vi "Sample--SaveandReadData.vi"() -> ()   [LabVIEW 2013]
doc: "This samples demonstrates how to sample a finite waveform."
uses:
  <userlib>/ArtScope/Trigger/ArtScope_ConfigureTriggerSoftWare.vi
  <userlib>/ArtScope/Fetch/ArtScope_FetchVoltage.vi
  <userlib>/ArtScope/Fetch/ArtScope_FetchBinary16.vi
panel:
  out "error out":errorcluster
  in  "reference position":dbl=100.0
  in  "DataType":i32(ring) items=["U8", "U16", "Voltage"]
  in  "range(Vpp)":i32(ring)=1 items=["20V", "10V", "2V", "40V", "16V", "8V", "4V", "1.6V", "800m", "400m", "160m", "80m", "40m"]
  out "waveform":dbl[][](graph)
  in  "ReadLength":i32=512
  out "waveform":dbl[][](graph)
  in  "FileName":string="D:\\1.PCI"
  in  "MinRecordLength":i32=60000
  in  "MinSampleRate":dbl=800000.0
  in  "Coupling":i32(ring) items=["DC", "AC"]
  in  "Channel Name":string="0"
  in  "Resource Name":string="Dev1"
  # "Vertical"
  # "Horizontal"
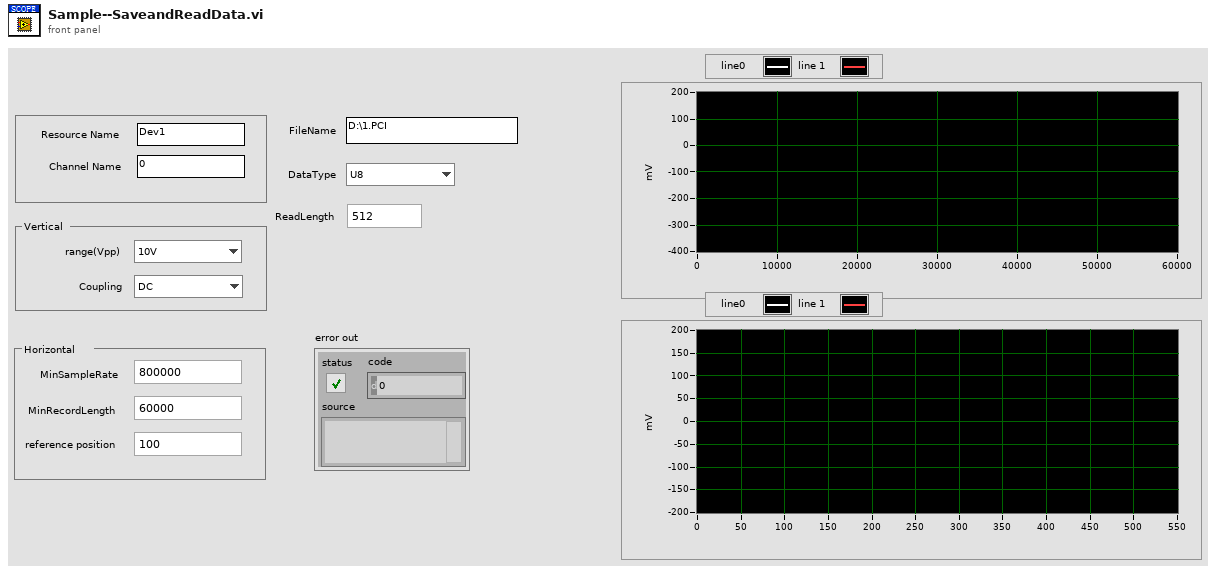
[diagram p1: front panel]
types:
  T1 = enum16{"big-endian, network order", "native, host order", "little-endian"}
  T2 = enum16{"open", "replace", "create", "open or create", "replace or create", "replace or create with confirmation"}
  T3 = cluster{"fLSB":cluster{dbl, dbl, dbl, dbl, dbl, dbl, dbl, dbl}, "RangeValue":cluster{dbl, dbl, dbl, dbl, dbl, dbl, dbl, dbl}, "wMaxLSB":u32, "TriggerMode":i32, "sampLengthPerChan":u32, "pAvailSampsPoints":u32, "channelCount":i32}
  T4 = cluster{"fLsbs":cluster{dbl, dbl, dbl, dbl, dbl, dbl, dbl, dbl}, "RangeValue":cluster{dbl, dbl, dbl, dbl, dbl, dbl, dbl, dbl}, "wMaxLSB":u32, "TriggerMode":i32, "actualSamples":u32, "pAvailSampsPoints":u32, "channelCount":i32}
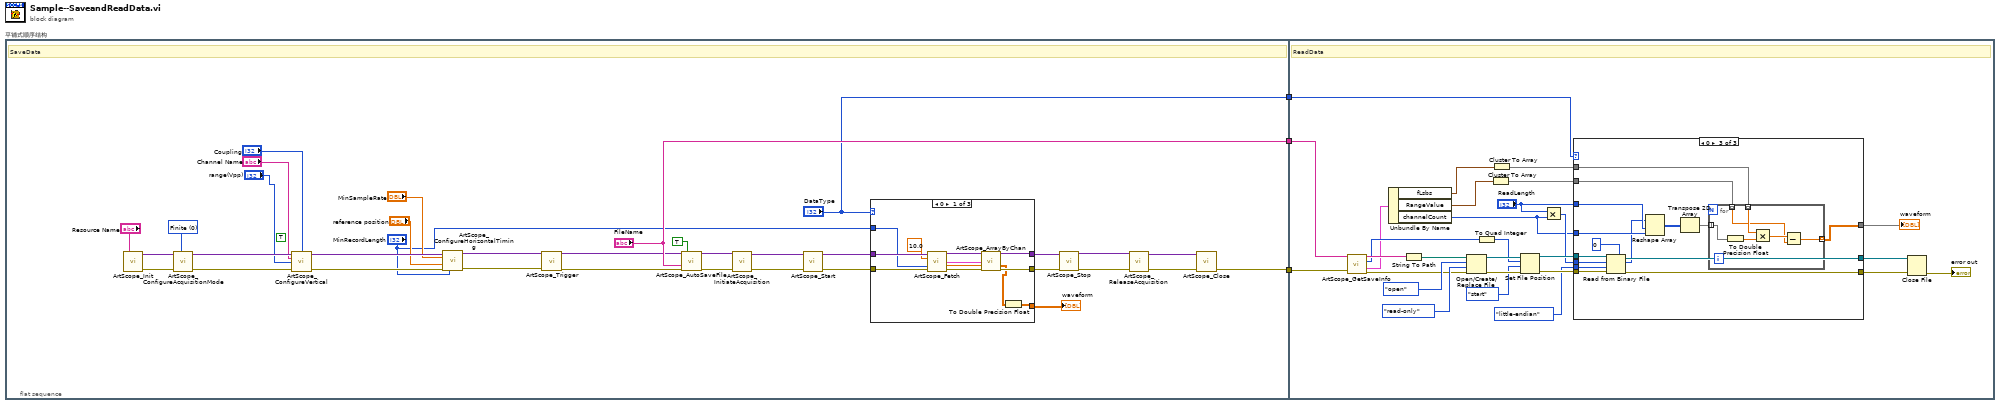
[diagram p0: block diagram]
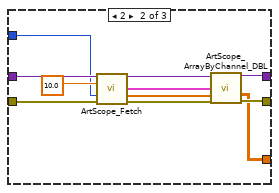
[diagram p2: hidden frame]
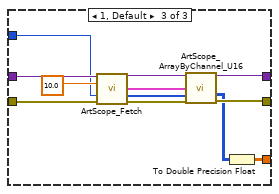
[diagram p3: hidden frame]
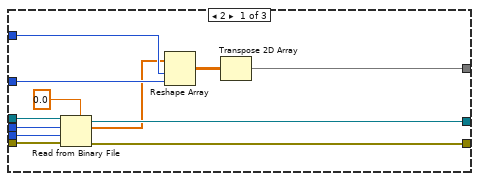
[diagram p4: hidden frame]
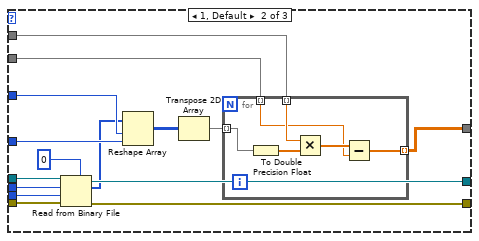
[diagram p5: hidden frame]
diagram:
  n1 = flat-sequence "平铺式顺序结构" {
    tunnel: ["FileName"] -> w3
    tunnel: [w10] -> w2
    tunnel: ["DataType"] -> w1
    tunnel: w3 -> [w99]
    tunnel: w2 -> [w98]
    tunnel: w1 -> [w79]
    frame #0 {
      (unwired) TRUE ("Enable")
      w30 = 0 items=["Finite", "Continuous"] ("AcuqMode")
      # "SaveData"
      n2 = call <userlib>:"ArtScope_Init.vi"("task name"="Resource Name") -> ("task handle"=w31:variant, "error out"=w32:errorcluster)  [unwired: 13 in]
      n3 = call <userlib>:"ArtScope_ConfigureAcquisitionMode.vi"("task handle"=w31, "acquisition mode"=w30, "error in (no error)"=w32) -> ("task handle"=w29:variant, "error out"=w33:errorcluster)  [unwired: 11 in]
      n4 = call <userlib>:"ArtScope_ConfigureVertical.vi"("task handle"=w29, "coupling"="Coupling", "channels"="Channel Name", "range(Vpp)"="range(Vpp)", "error in (no error)"=w33) -> ("task handle"=w35:variant, "error out"=w34:errorcluster)  [unwired: 9 in]
      n5 = call <userlib>:"ArtScope_ConfigureHorizontalTiming.vi"("task handle"=w35, "min sample rate"="MinSampleRate", "reference position"="reference position", "error in (no error)"=w34, "min record length"="MinRecordLength") -> ("task handle"=w27:variant, "error out"=w28:errorcluster)  [unwired: 9 in]
      n6 = call-poly <userlib>:"ArtScope_Trigger.vi"("task handle"=w27, "error in (no error)"=w28) -> ("task handle"=w17:variant, "error out"=w16:errorcluster)  [unwired: 12 in]
      n7 = call <userlib>:"ArtScope_AutoSaveFile.vi"("task handle"=w17, "auto save"=TRUE ("AutoSave"), "file name"="FileName", "error in (no error)"=w16) -> ("task handle"=w14:variant, "error out"=w15:errorcluster)  [unwired: 10 in]
      n8 = call <userlib>:"ArtScope_InitiateAcquisition.vi"("task handle"=w14, "error in (no error)"=w15) -> ("task handle"=w23:variant, "error out"=w22:errorcluster)  [unwired: 12 in]
      n9 = call <userlib>:"ArtScope_Start.vi"("task handle"=w23, "error in (no error)"=w22) -> ("task handle"=w9:variant, "error out"=w8:errorcluster)  [unwired: 12 in]
      n10 = case shown="0" "DataType" {
        tunnel: [w45 w56 w68] -> w12
        tunnel: [w44 w54 w67] -> w11
        tunnel: w9 -> [w50 w61 w73]
        tunnel: w8 -> [w49 w60 w72]
        tunnel: "MinRecordLength" -> [w47 w58 w70]
        tunnel: [w40 w51 w63] -> w5
        frame 0 {
          n11 = call-poly <userlib>:"ArtScope_Fetch.vi"("task handle"=w50, "timeout"=10.0, "num samples"=w47, "error in (no error)"=w49) -> ("task handle"=w43:variant, "wfm info"=w42:T3, "data"=w41:dbl[], "error out"=w46:errorcluster)  [unwired: 8 in]
          n12 = call-poly <userlib>:"ArtScope_ArrayByChan.vi"("task handle"=w43, "wfm info"=w42, "1D data"=w41, "error in (no error)"=w46) -> ("task handle"=w44:variant, "2D data"=w39:dbl[][], "error out"=w45:errorcluster)  [unwired: 9 in]
          n13 = To Double Precision Float(number=w39) -> (double precision float=w40:dbl[][])
        }
        frame 2 {
          n14 = call-poly <userlib>:"ArtScope_Fetch.vi"("task handle"=w61, "timeout"=10.0 ("Timeout(s)"), "num samples"=w58, "error in (no error)"=w60) -> ("task handle"=w55:variant, "wfm info"=w53:T3, "data"=w52:dbl[], "error out"=w57:errorcluster)  [unwired: 8 in]
          n15 = call <userlib>:"ArtScope_ArrayByChannel_DBL.vi"("task handle"=w55, "wfm info"=w53, "1D data"=w52, "error in (no error)"=w57) -> ("task handle"=w54:variant, "2D data"=w51:dbl[][], "error out"=w56:errorcluster)  [unwired: 9 in]
        }
        frame 1, Default {
          n16 = call-poly <userlib>:"ArtScope_Fetch.vi"("task handle"=w73, "timeout"=10.0 ("Timeout(s)"), "num samples"=w70, "error in (no error)"=w72) -> ("task handle"=w66:variant, "wfm info"=w64:T3, "data"=w65:u16[], "error out"=w69:errorcluster)  [unwired: 8 in]
          n17 = call <userlib>:"ArtScope_ArrayByChannel_U16.vi"("task handle"=w66, "wfm info"=w64, "1D data"=w65, "error in (no error)"=w69) -> ("task handle"=w67:variant, "2D data"=w62:u16[][], "error out"=w68:errorcluster)  [unwired: 9 in]
          n18 = To Double Precision Float(number=w62) -> (double precision float=w63:dbl[][])
        }
      }
      "waveform" <- w5
      n19 = call <userlib>:"ArtScope_Stop.vi"("task handle"=w11, "error in (no error)"=w12) -> ("task handle"=w21:variant, "error out"=w20:errorcluster)  [unwired: 12 in]
      n20 = call <userlib>:"ArtScope_ReleaseAcquisition.vi"("task handle"=w21, "error in (no error)"=w20) -> ("task handle"=w19:variant, "error out"=w18:errorcluster)  [unwired: 12 in]
      n21 = call <userlib>:"ArtScope_Close.vi"("task handle"=w19, "error in (no error)"=w18) -> ("error out"=w10:errorcluster)  [unwired: 13 in]
    }
    frame #1 {
      # "ReadData"
      n22 = call <userlib>:"ArtScope_GetSaveInfo.vi"("file name"=w99, "error in (no error)"=w98) -> ("file name"=w95:string, "header size"=w92:i32, "file wfm info"=w87:T4, "error out"=w97:errorcluster)  [unwired: 10 in]
      n23 = Unbundle By Name(w87) -> ("fLsbs"=w78:cluster{dbl, dbl, dbl, dbl, dbl, dbl, dbl, dbl}, "RangeValue"=w76:cluster{dbl, dbl, dbl, dbl, dbl, dbl, dbl, dbl}, "channelCount"=w83:i32)
      n24 = String To Path(string=w95) -> (path=w96:path)
      n25 = Open/Create/Replace File(file path (use dialog)=w96, error in=w97, operation (0:open)=T2."open" ("操作(0:open)"), access (0:read/write)=enum16{"read/write", "read-only", "write-only"}."read-only" ("权限(0:read/write)")) -> (refnum out=w94:refnum<file>, error out=w93:errorcluster)  [unwired: 2 in, 1 out]
      n26 = To Quad Integer(1:w92) -> (0:w91:i64)
      n27 = Cluster To Array(cluster=w76) -> (array=w75:dbl[])
      n28 = Cluster To Array(cluster=w78) -> (array=w77:dbl[])
      n29 = Set File Position(offset (in bytes) (0)=w91, refnum=w94, from (0:start)=enum16{"start", "end", "current"}."start" ("自（0:起始）"), error in=w93) -> (refnum out=w89:refnum<file>, error out=w88:errorcluster)
      n30 = Multiply(x="ReadLength", y=w83) -> (x*y=w86:i32)
      n31 = case shown="0" w79 {
        tunnel: w89 -> [w113 w128 w149]
        tunnel: w88 -> [w112 w127 w148]
        tunnel: w86 -> [w111 w126 w147]
        tunnel: T1."little-endian" ("字节顺序(0:big-endian, network order)") -> [w110 w125 w146]
        tunnel: "ReadLength" -> [w109 w124 w145]
        tunnel: w83 -> [w108 w123 w144]
        tunnel: [w106 w114 w135] -> w82
        tunnel: [w105 w121 w142] -> w81
        tunnel: [w104 w120 w141] -> w80
        tunnel: w77 -> [_ w116 w137]
        tunnel: w75 -> [_ w115 w136]
        frame 2 {
          n32 = Read from Binary File(5:0.0, 8:w112, 9:w110, 10:w111, 11:w113) -> (0:w105:errorcluster, 2:w102:dbl[], 3:w104:refnum<file>)  [unwired: 1 in, 1 out]
          n33 = Reshape Array(w102, w109, w108) -> (w107:dbl[][])
          n34 = Transpose 2D Array(2D array=w107) -> (transposed array=w106:dbl[][])
        }
        frame 1, Default {
          n35 = Read from Binary File(5:u16 0, 8:w127, 9:w125, 10:w126, 11:w128) -> (0:w121:errorcluster, 2:w118:u16[], 3:w120:refnum<file>)  [unwired: 1 in, 1 out]
          n36 = Reshape Array(w118, w124, w123) -> (w122:u16[][])
          n37 = Transpose 2D Array(2D array=w122) -> (transposed array=w117:u16[][])
          n38 = for {
            tunnel: w117 -> [w129] mode=indexing
            tunnel: w115 -> [w131] mode=indexing
            tunnel: w116 -> [w134] mode=indexing
            tunnel: [w130] -> w114 mode=indexing
            n39 = To Double Precision Float(number=w129) -> (double precision float=w133:dbl[])
            n40 = Multiply(x=w134, y=w133) -> (x*y=w132:dbl[])
            n41 = Subtract(x=w132, y=w131) -> (x-y=w130:dbl[])
          }
        }
        frame 0 {
          n42 = Read from Binary File(5:u8 0, 8:w148, 9:w146, 10:w147, 11:w149) -> (0:w142:errorcluster, 2:w139:u8[], 3:w141:refnum<file>)  [unwired: 1 in, 1 out]
          n43 = Reshape Array(w139, w145, w144) -> (w143:u8[][])
          n44 = Transpose 2D Array(2D array=w143) -> (transposed array=w138:u8[][])
          n45 = for {
            tunnel: w138 -> [w150] mode=indexing
            tunnel: w136 -> [w152] mode=indexing
            tunnel: w137 -> [w155] mode=indexing
            tunnel: [w151] -> w135 mode=indexing
            n46 = To Double Precision Float(number=w150) -> (double precision float=w154:dbl[])
            n47 = Multiply(x=w155, y=w154) -> (x*y=w153:dbl[])
            n48 = Subtract(x=w153, y=w152) -> (x-y=w151:dbl[])
          }
        }
      }
      "waveform" <- w82
      n49 = Close File(refnum=w80, error in=w81) -> (error out=→"error out":errorcluster)  [unwired: 1 out]
    }
  }
